vi "PythonConfiguration.vi"(8 "error in":errorcluster, 11 "Configuration Path":path) -> (0 "error out":errorcluster, 3 "PythonConfiguration out":refnum<class "PythonConfiguration.lvclass">)   [LabVIEW 2014, in "Raspberry Pi Compatible Compiler for LabVIEW.lvlib" / "PythonConfiguration.lvclass"]
uses:
  PythonConfiguration.lvclass
  PythonConfiguration.lvclass/PythonConfiguration.ctl
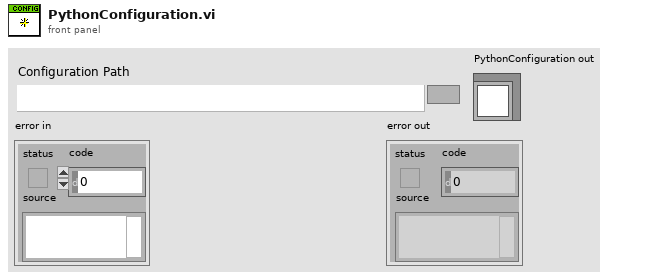
[diagram p1: front panel]
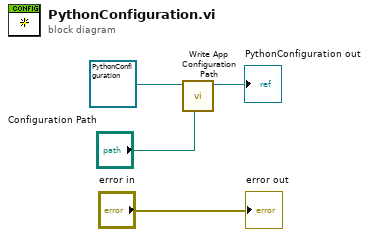
[diagram p0: block diagram]
diagram:
  n1 = call "Write App Configuration Path.vi"("App Configuration Path"="Configuration Path", "PythonConfiguration in"=refnum<class "PythonConfiguration.lvclass"> refnum) -> ("PythonConfiguration out"=→"PythonConfiguration out":refnum<class "PythonConfiguration.lvclass">)  [unwired: 7 in]
  "error out" <- "error in"
